vi "Write Multiple Registers Request.vi"(8 "error in":errorcluster, 9 "Registers":u16[](array[numeric]), 10 "Starting Address":u16) -> (0 "error out":errorcluster, 2 "modbus data unit out":refnum<class "Modbus Data Unit.lvclass">)   [LabVIEW 2013, in "Modbus Library - Advance.lvlib" / "Master Function Definition.lvclass"]
doc: "This VI forms a modbus data unit for writing multiple registers."
uses:
  Master Function Definition.lvclass
  Modbus Data Unit/Modbus Data Unit.lvclass
  Modbus Data Unit/Function.ctl
  Modbus Data Unit/Modbus Data Unit.lvclass/Modbus Data Unit.ctl
  Modbus Library - Advance.lvlib
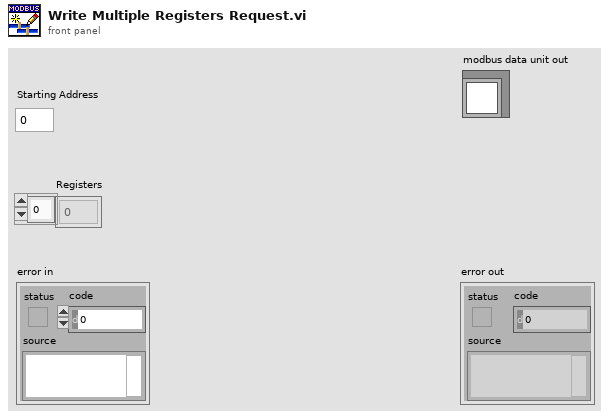
[diagram p1: front panel]
types:
  T1 = typedef "Modbus Library - Advance.lvlib/Modbus Data Unit.lvclass/Function.ctl" = u8
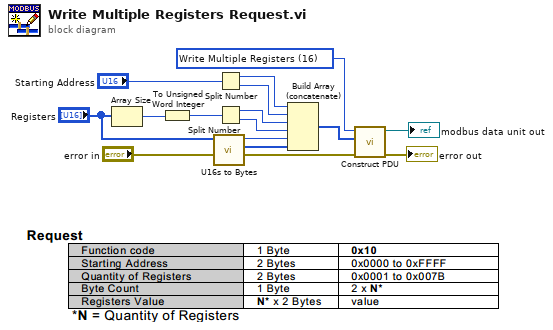
[diagram p0: block diagram]
diagram:
  w6 = T1 16 items=["Read Discrete Inputs"=2, "Read Coils"=1, "Write Single Coil"=5, "Write Multiple Coils"=15, "Read Input Register"=4, "Read Holding Registers"=3, "Write Single Register"=6, "Write Multiple Registers"=16, "Read/Write Multiple Registers"=23, "Mask Write Register"=22, "Read FIFO Queue"=24, "Read File Record"=20, "Write File Record"=21, "Read Exception Status"=7, "Diagnostic"=8, "Get Com Event Counter"=11, "Get Com Event Log"=12, "Report Slave ID"=17, "Read Device Identification"=43] ("Function")
  n1 = Array Size(array="Registers") -> (size(s)=w4:i32)
  n2 = To Unsigned Word Integer(number=w4) -> (unsigned 16bit integer=w3:u16)
  n3 = call "U16s to Bytes.vi"("Registers"="Registers") -> ("Bytes"=w1:u8[], "Count"=w2:u8)  [unwired: 9 in]
  n4 = Split Number(x="Starting Address") -> (hi(x)=w8:u8, lo(x)=w9:u8)
  n5 = Split Number(x=w3) -> (hi(x)=w10:u8, lo(x)=w11:u8)
  n6 = Build Array (concatenate)(w8, w9, w10, w11, w2, w1) -> (w7:u8[])
  n7 = call "Construct PDU.vi"("error in"="error in", "data"=w7, "Function"=w6) -> ("error out"=→"error out":errorcluster, "modbus data unit out"=→"modbus data unit out":refnum<class "Modbus Data Unit.lvclass">)  [unwired: 7 in]
